vi "Start Log.vi"(8 "error in (no error)":errorcluster, 9 "Timestamp":string, 10 "Series":string, 11 "DataLogger in":refnum<class "DataLogger.lvclass">) -> (0 "error out":errorcluster, 3 "DataLogger out":refnum<class "DataLogger.lvclass">)   [LabVIEW 2020, in "VolatusDataLogger.lvlib" / "DataLogger.lvclass"]
uses:
  DataLogger.lvclass
  DataLogger.lvclass/DataLogger.ctl
  Volatus/Task/Task.lvclass
  C:/dev/lv20CE/relink/lv-volatus/Volatus/Task/Task.lvclass
  C:/Program Files (x86)/National Instruments/LabVIEW 2020/vi.lib/ActorFramework/Actor/Actor.lvclass
  C:/dev/lv20CE/relink/lv-volatus/Volatus/APIRegistrationHandler/APIRegistrationHandler.lvclass
  C:/dev/lv20CE/relink/lv-volatus/Volatus/TaskStateHandler/TaskStateHandler.lvclass
  C:/dev/lv20CE/relink/lv-volatus/Volatus/VectoMessageHandler/VectoMessageHandler.lvclass
  C:/dev/lv20CE/relink/lv-volatus/VolatusDataLogger/DataLogger/DataLogger.lvclass
  C:/dev/lv20CE/relink/lv-volatus/Volatus/API Provider/API Provider.lvclass
  C:/dev/lv20CE/relink/lv-volatus/VolatusDataLogger/LoggingHandler/LoggingHandler.lvclass
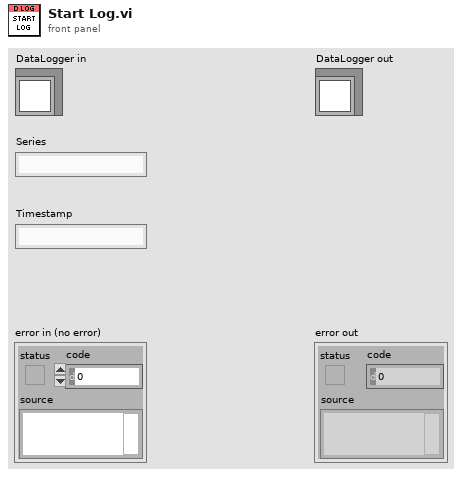
[diagram p1: front panel]
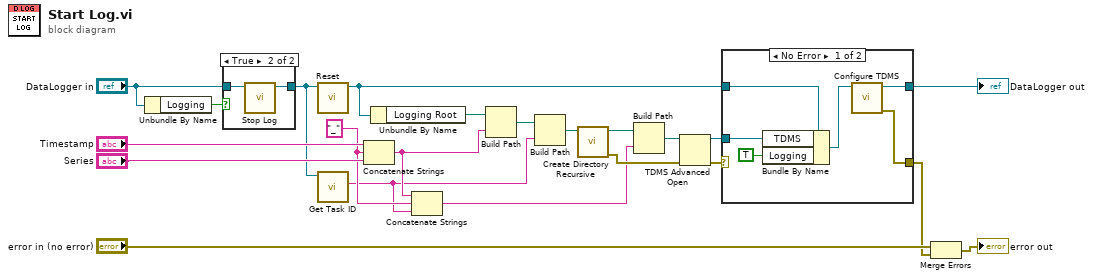
[diagram p0: block diagram]
diagram:
  w11 = "_" ("string")
  n1 = Unbundle By Name("DataLogger in") -> ("Logging"=w1:bool)
  n2 = case shown="True" w1 {
    tunnel: "DataLogger in" -> [w23 w25]
    tunnel: [w23 w24] -> w2
    frame False {
    }
    frame True {
      n3 = call-dynamic "Stop Log.vi"("DataLogger in"=w25) -> ("DataLogger out"=w24:refnum<class "DataLogger.lvclass">)  [unwired: 9 in, 1 out]
    }
  }
  n4 = call "Reset.vi"("DataLogger in"=w2) -> ("DataLogger out"=w6:refnum<class "DataLogger.lvclass">)  [unwired: 9 in, 1 out]
  n5 = call "Get Task ID.vi"("Task in"=w2) -> ("Task ID"=w10:string)  [unwired: 9 in, 1 out]
  n6 = Concatenate Strings("Timestamp", w11, "Series") -> (w12:string)
  n7 = Unbundle By Name(w6) -> ("Logging Root"=w15:path)
  n8 = Concatenate Strings(w12, w11, w10) -> (w8:string)
  n9 = Build Path(base path=w15, name or relative path=w12) -> (appended path=w14:path)
  n10 = Build Path(base path=w14, name or relative path=w10) -> (appended path=w13:path)
  n11 = call <vilib>:"Create Directory Recursive.vi"("directory"=w13) -> ("error out"=w16:errorcluster, "directory copy"=w9:path)  [unwired: 4 in, 1 out]
  n12 = Build Path(base path=w9, name or relative path=w8) -> (appended path=w7:path)
  n13 = TDMS Advanced Open(8:w16, 11:w7) -> (0:w4:errorcluster, 3:w5:refnum<k34>)  [unwired: 3 in, 1 out]
  n14 = case shown="No Error" w4 {
    selector: w4 -> [_ w33]
    tunnel: w6 -> [w31 w32]
    tunnel: w5 -> [w30 _]
    tunnel: [w27 w32] -> w18
    tunnel: [w26 w33] -> w3
    frame No Error {
      n15 = Bundle By Name(cluster=w31, "TDMS"=w30, "Logging"=TRUE) -> (w28:refnum<class "DataLogger.lvclass">)
      n16 = call "Configure TDMS.vi"("DataLogger in"=w28) -> ("error out"=w26:errorcluster, "DataLogger out"=w27:refnum<class "DataLogger.lvclass">)  [unwired: 9 in]
    }
    frame Error {
    }
  }
  "DataLogger out" <- w18
  n17 = Merge Errors("error in (no error)", w3) -> (→"error out":errorcluster)
